vi "getFPGAReference.vi"(11 "FPGATelemetry in":refnum<class "RTHealthAndStatus.lvclass">) -> (2 "FPGAReference":refnum<k20>, 3 "FPGATelemetry out":refnum<class "RTHealthAndStatus.lvclass">)   [LabVIEW 2015]
uses:
  RTHealthAndStatus.lvclass
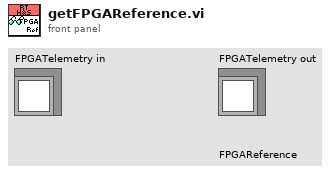
[diagram p1: front panel]
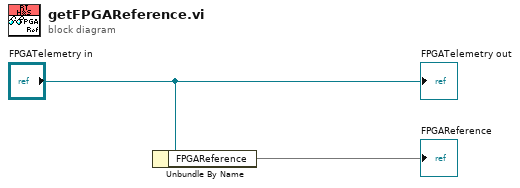
[diagram p0: block diagram]
diagram:
  n1 = Unbundle By Name("FPGATelemetry in") -> ("FPGAReference"=→"FPGAReference")
  "FPGATelemetry out" <- "FPGATelemetry in"
